vi "toStringArray.vi"(8 "error in (no error)":errorcluster, 11 "RampToneUp in":refnum<class "RampToneUp.lvclass">) -> (0 "error out":errorcluster, 2 "eventStringArray":string[](array[string]), 3 "RampToneUp out":refnum<class "RampToneUp.lvclass">)   [LabVIEW 2011, in "Tools.lvlib" / "Scripting.lvlib" / "RampToneUp.lvclass"]
uses:
  RampToneUp.lvclass
  RampTone/RampTone.lvclass
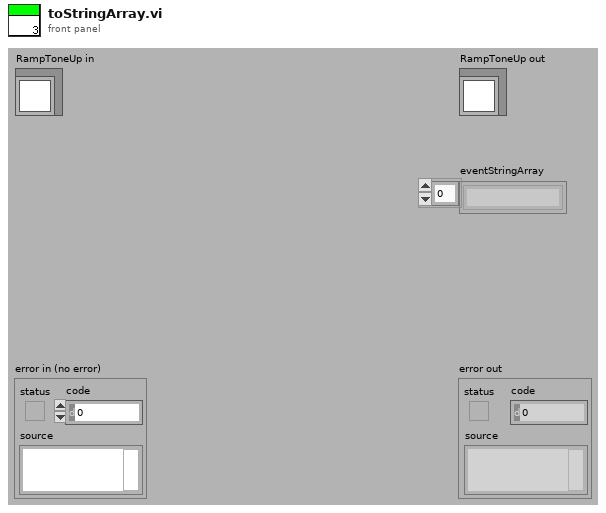
[diagram p1: front panel]
types:
  T1 = cluster{"rampTime":dbl, "timeStep":dbl, "dataValueStep":dbl}
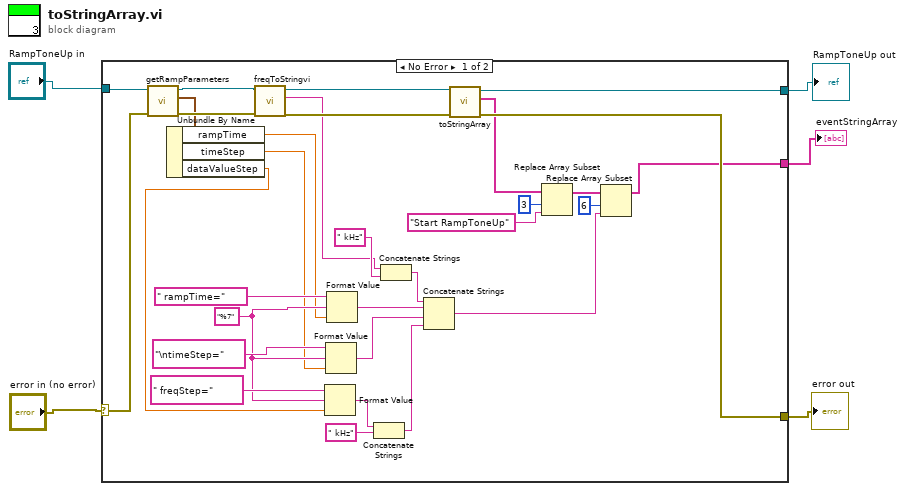
[diagram p0: block diagram]
diagram:
  n1 = case shown="No Error" "error in (no error)" {
    selector: "error in (no error)" -> [w11 w37]
    tunnel: [w36 w37] -> w5
    tunnel: [w21 _] -> w4
    tunnel: "RampToneUp in" -> [w12 w38]
    tunnel: [w20 w38] -> w1
    frame No Error {
      w19 = "%7"
      n2 = call "getRampParameters.vi"("error in (no error)"=w11, "RampTone in"=w12) -> ("error out"=w10:errorcluster, "RampParameters"=w9:T1, "RampTone out"=w13:refnum<class "RampToneUp.lvclass">)  [unwired: 7 in]
      n3 = Unbundle By Name(w9) -> ("rampTime"=w8:dbl, "timeStep"=w7:dbl, "dataValueStep"=w6:dbl)
      n4 = call-dynamic "freqToStringvi.vi"("error in (no error)"=w10, "SingleTone in"=w13) -> ("error out"=w17:errorcluster, "frequency"=w14:string, "SingleTone out"=w18:refnum<class "RampToneUp.lvclass">)  [unwired: 7 in]
      n5 = Format Value(string ("")=" freqStep=", format string=w19, value (0)=w6) -> (output string=w24:string)
      n6 = Format Value(string ("")="\ntimeStep=", format string=w19, value (0)=w7) -> (output string=w27:string)
      n7 = Format Value(string ("")=" rampTime=", format string=w19, value (0)=w8) -> (output string=w28:string)
      n8 = Concatenate Strings(w24, " kHz") -> (w22:string)
      n9 = Concatenate Strings(w14, " kHz") -> (w15:string)
      n10 = Concatenate Strings(w15, w28, w27, w22) -> (w26:string)
      n11 = call-parent "toStringArray.vi"("error in (no error)"=w17, "RampTone in"=w18) -> ("error out"=w36:errorcluster, "eventStringArray"=w25:string[], "RampTone out"=w20:refnum<class "RampToneUp.lvclass">)  [unwired: 7 in]
      n12 = Replace Array Subset(array=w25, new element="Start RampToneUp", index=3) -> (w31:string[])
      n13 = Replace Array Subset(array=w31, new element=w26, index=6) -> (w21:string[])
    }
    frame Error {
    }
  }
  "error out" <- w5
  "RampToneUp out" <- w1
  "eventStringArray" <- w4
